vi "output.vi"(8 "error in":errorcluster, 10 "data table in":T1, 11 "JSON_RPC_Interface runtime in":refnum<class "JSON_RPC_Interface runtime.lvclass">) -> (0 "error out":errorcluster, 2 "data table out":T1, 3 "JSON_RPC_Interface runtime out":refnum<class "JSON_RPC_Interface runtime.lvclass">)   [LabVIEW 2017, in "JSON_RPC_Interface runtime.lvclass"]
doc: "Provides an interface for writing data to a module at runtime. While this interface performs no operations, a child should provide an override which may write to any open sessions, references, or interfaces."
uses:
  JSON_RPC_Interface runtime.lvclass
  <vilib>/NI/Tag Bus/table/data table.ctl
  JSON_RPC_Interface runtime.lvclass/JSON_RPC_Interface runtime.ctl
  <vilib>/NI/NI JSONRPC Server Framework/Classes/Request/Request.lvclass/Request.ctl
  <vilib>/NI/Tag Bus/table/data polymorphs/read one/read Double.vi
  <vilib>/NI/Tag Bus/table/data polymorphs/read one/read Single.vi
  <vilib>/NI/Tag Bus/table/data polymorphs/read one/read I64.vi
  <vilib>/NI/Tag Bus/table/data polymorphs/read one/read I32.vi
  <vilib>/NI/Tag Bus/table/data polymorphs/read one/read I16.vi
  <vilib>/NI/Tag Bus/table/data polymorphs/read one/read I8.vi
  <vilib>/NI/Tag Bus/table/data polymorphs/read one/read U64.vi
  <vilib>/NI/Tag Bus/table/data polymorphs/read one/read U32.vi
  <vilib>/NI/Tag Bus/table/data polymorphs/read one/read U16.vi
  <vilib>/NI/Tag Bus/table/data polymorphs/read one/read U8.vi
  <vilib>/NI/Tag Bus/table/data polymorphs/read one/read Boolean.vi
  <vilib>/NI/Tag Bus/table/data polymorphs/read one/read String.vi
  <vilib>/NI/Tag Bus/table/data polymorphs/read one/read Array of Double.vi
  <vilib>/NI/Tag Bus/table/data polymorphs/read one/read Array of Single.vi
  <vilib>/NI/Tag Bus/table/data polymorphs/read one/read Array of I64.vi
  <vilib>/NI/Tag Bus/table/data polymorphs/read one/read Array of I32.vi
  <vilib>/NI/Tag Bus/table/data polymorphs/read one/read Array of I16.vi
  <vilib>/NI/Tag Bus/table/data polymorphs/read one/read Array of I8.vi
  <vilib>/NI/Tag Bus/table/data polymorphs/read one/read Array of U64.vi
  <vilib>/NI/Tag Bus/table/data polymorphs/read one/read Array of U32.vi
  <vilib>/NI/Tag Bus/table/data polymorphs/read one/read Array of U16.vi
  <vilib>/NI/Tag Bus/table/data polymorphs/read one/read Array of U8.vi
  <vilib>/NI/Tag Bus/table/data polymorphs/read one/read Array of Boolean.vi
  <vilib>/NI/Tag Bus/table/data polymorphs/read one/read Array of String.vi
  <vilib>/NI/NI JSONRPC Server Framework/Classes/Request/request.Read params.vi
  <vilib>/NI/NI JSONRPC Server Framework/Classes/params/params.To JSON Tree.vi
  <vilib>/NI/NI JSONRPC Server Framework/Classes/Server/Add Response (Internal Error from Request).vi
  <vilib>/NI/JSON Support for LabVIEW/JSON Value/New JSON Value/New JSON ({String}).vi
  <vilib>/NI/NI JSONRPC Server Framework/Classes/Server/Add Response (Invalid Params from Request).vi
  <vilib>/NI/JSON Support for LabVIEW/JSON Value/Object/Insert Value/Insert Value (Numeric).vi
  <vilib>/NI/JSON Support for LabVIEW/JSON Value/Object/Insert Value/Insert Value (Boolean).vi
  <vilib>/NI/JSON Support for LabVIEW/JSON Value/Object/Insert Value/Insert Value (String).vi
  <vilib>/NI/JSON Support for LabVIEW/JSON Value/Object/Insert Value/Insert Value (Numeric[]).vi
  <vilib>/NI/JSON Support for LabVIEW/JSON Value/Object/Insert Value/Insert Value (Boolean[]).vi
  <vilib>/NI/JSON Support for LabVIEW/JSON Value/Object/Insert Value/Insert Value (String[]).vi
  <vilib>/NI/NI JSONRPC Server Framework/Classes/Server/Add Response (Result from Request).vi
  <vilib>/NI/JSON Support for LabVIEW/JSON Value/JSON Value.lvclass
  <vilib>/NI/Tag Bus/table/data table.lvlib
  <vilib>/NI/NI JSONRPC Server Framework/Classes/Server/JSONRPC Server.lvclass
  <vilib>/NI/NI JSONRPC Server Framework/Classes/Request/Request.lvclass
  <vilib>/NI/JSON Support for LabVIEW/JSON Variant Support/JSON Variant Support.lvclass
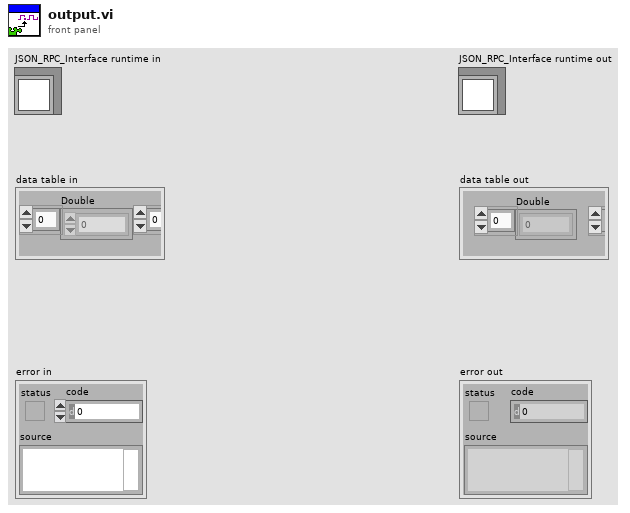
[diagram p1: front panel]
types:
  T1 = typedef "tag bus.lvlib/data table.lvlib/data table.ctl" = cluster{"Double":dbl[], "Single":sgl[], "I64":i64[], "I32":i32[], "I16":i16[], "I8":i8[], "U64":u64[], "U32":u32[], "U16":u16[], "U8":u8[], "Boolean":bool[], "String":string[], "Array of Double":cluster{"DBL Array":dbl[]}[], "Array of Single":cluster{"SGL Array":sgl[]}[], "Array of I64":cluster{"I64 Array":i64[]}[], "Array of I32":cluster{"I32 Array":i32[]}[], "Array of I16":cluster{"I16 Array":i16[]}[], "Array of I8":cluster{"I8 Array":i8[]}[], "Array of U64":cluster{"U64 Array":u64[]}[], "Array of U32":cluster{"U32 Array":u32[]}[], "Array of U16":cluster{"U16 Array":u16[]}[], "Array of U8":cluster{"U8 Array":u8[]}[], "Array of Boolean":cluster{"Boolean Array":bool[]}[], "Array of String":cluster{"String Array":string[]}[]}
  T2 = typedef "tag bus.lvlib/tag descriptor.lvclass/Data Type.ctl" = enum16{"Double", "Single", "I64", "I32", "I16", "I8", "U64", "U32", "U16", "U8", "Boolean", "String", "Array of Double", "Array of Single", "Array of I64", "Array of I32", "Array of I16", "Array of I8", "Array of U64", "Array of U32", "Array of U16", "Array of U8", "Array of Boolean", "Array of String"}
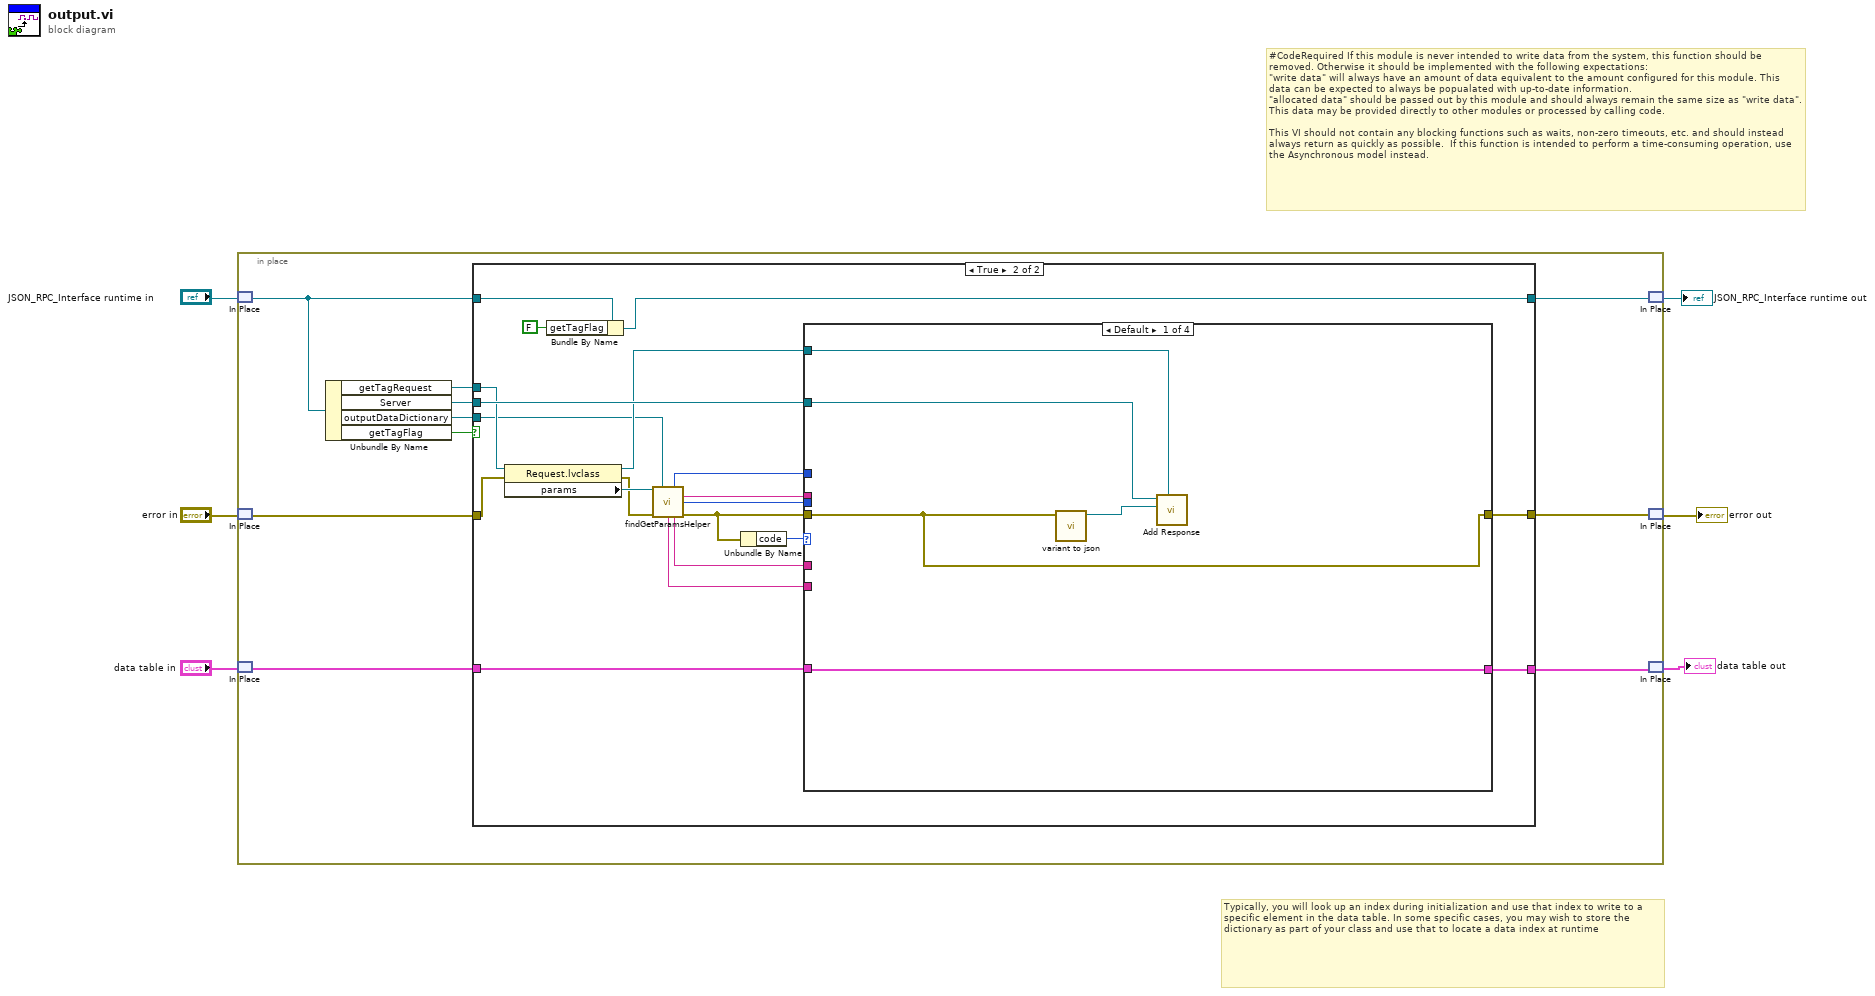
[diagram p0: block diagram]
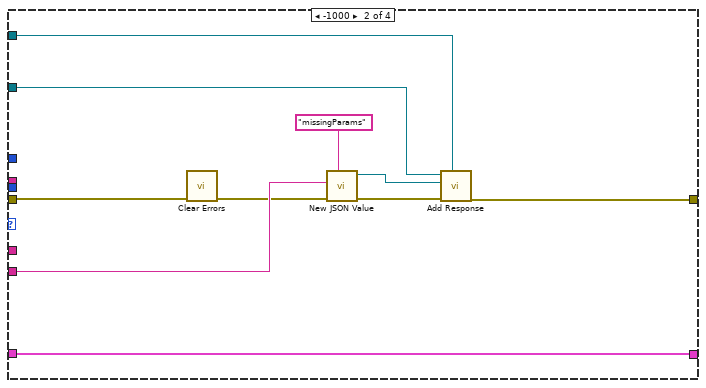
[diagram p3: hidden frame]
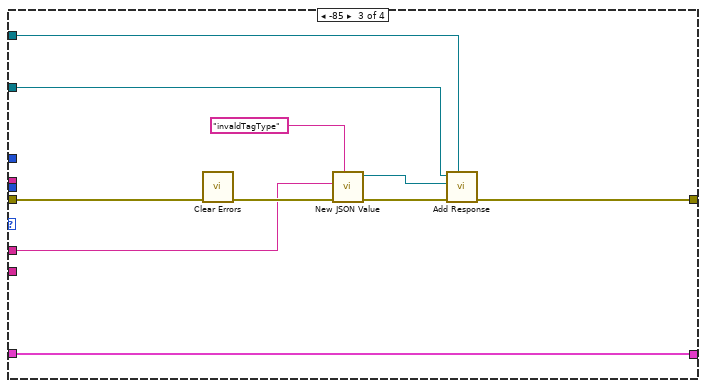
[diagram p4: hidden frame]
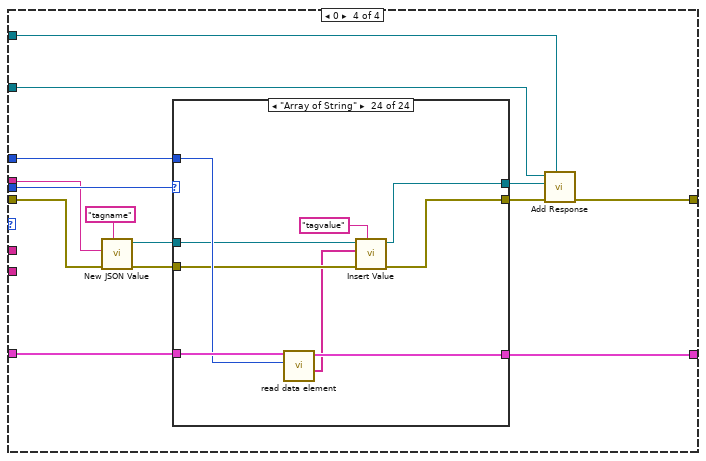
[diagram p5: hidden frame]
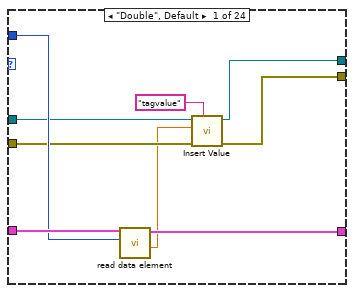
[diagram p6: hidden frame]
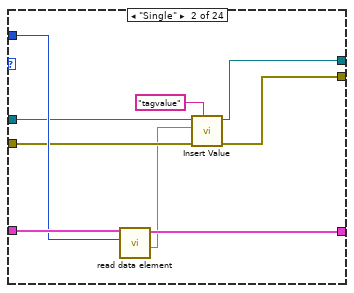
[diagram p7: hidden frame]
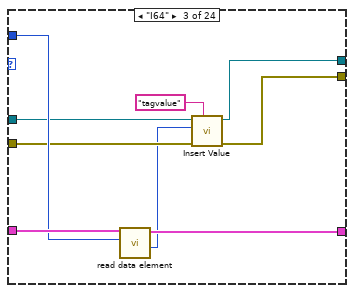
[diagram p8: hidden frame]
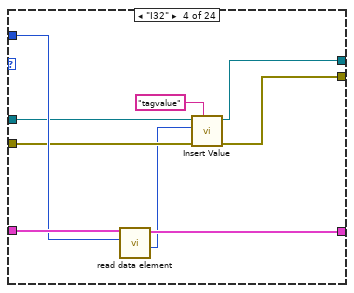
[diagram p9: hidden frame]
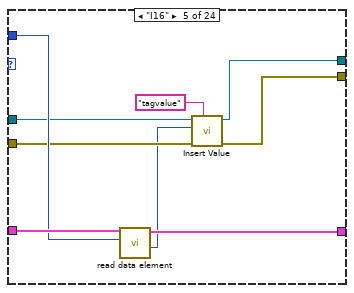
[diagram p10: hidden frame]
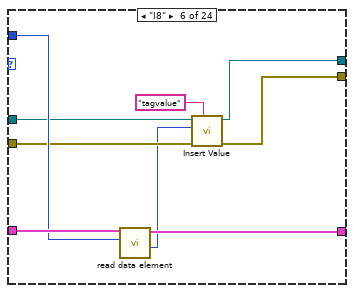
[diagram p11: hidden frame]
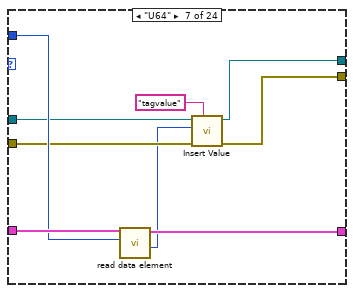
[diagram p12: hidden frame]
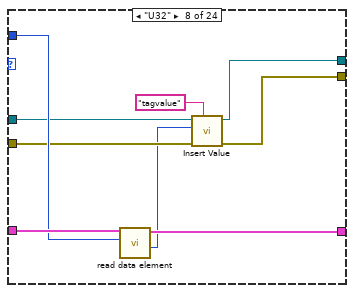
[diagram p13: hidden frame]
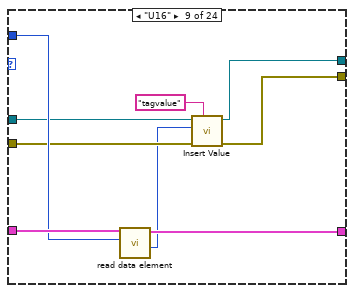
[diagram p14: hidden frame]
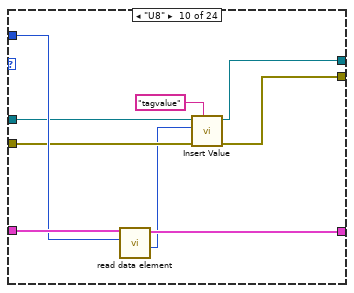
[diagram p15: hidden frame]
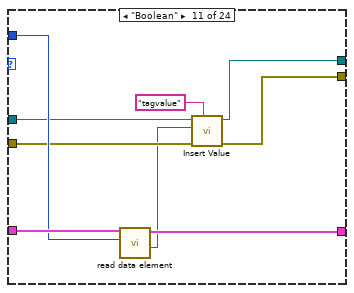
[diagram p16: hidden frame]
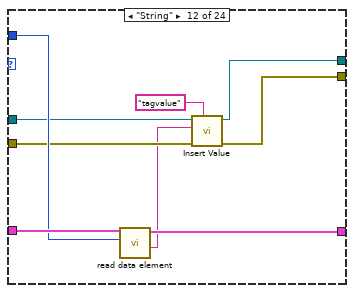
[diagram p17: hidden frame]
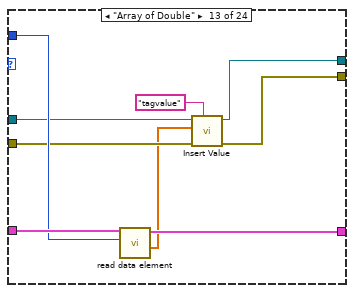
[diagram p18: hidden frame]
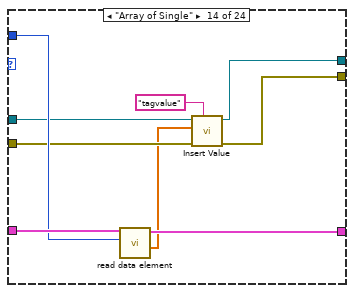
[diagram p19: hidden frame]
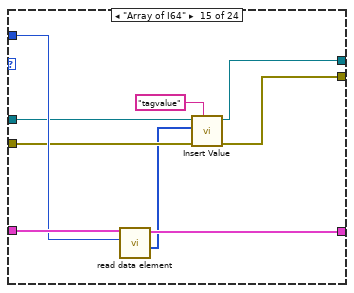
[diagram p20: hidden frame]
diagram:
  # "Typically, you will look up an index during initialization and use that index to write to a specific element in the data table. In some specific cases, you may wish to store the dictionary as part of your class and use that to locate a data index at runtime"
  # "#CodeRequired If this module is never intended to write data from the system, this function should be removed. Otherwise it should be implemented with the following expectations:\n\"write data\" will always have an amount of data equivalent to the amount configured for this module. This data can be expected to always be popualated with up-to-date information.\n\"allocated data\" should be passed out by this module and should always remain the same size as \"write data\". This data may be provided directly to other modules or processed by calling code.\n\nThis VI should not contain any blocking functions such as waits, non-zero timeouts, etc. and should instead always return as quickly as possible.  If this function is intended to perform a time-consuming operation, use the Asynchronous model instead."
  n1 = in-place {
    n2 = in-place-match #1("JSON_RPC_Interface runtime in") -> (w8:refnum<class "JSON_RPC_Interface runtime.lvclass">)
    n3 = in-place-match #2("error in") -> (w11:errorcluster)
    n4 = in-place-match #3("data table in") -> (w16:T1)
    n5 = Unbundle By Name(w8) -> ("getTagRequest"=w12:refnum<class "Request.lvclass">, "Server"=w13:refnum<class "JSONRPC Server.lvclass">, "outputDataDictionary"=w10:refnum<class "data dictionary.lvclass">, "getTagFlag"=w9:bool)
    n6 = case shown="True" w9 {
      tunnel: w16 -> [w19 w38]
      tunnel: [w19 w37] -> w15
      tunnel: [w18 w36] -> w14
      tunnel: w13 -> [_ w35]
      tunnel: w12 -> [_ w34]
      tunnel: w11 -> [w18 w32]
      tunnel: w10 -> [_ w30]
      tunnel: w8 -> [w17 w22]
      tunnel: [w17 w20] -> w7
      frame False {
      }
      frame True {
        n7 = property class="Request.lvclass"(reference=w34, error in=w32) -> (reference out=w33:refnum<class "Request.lvclass">, error out=w29:errorcluster, "params"=w31:refnum<class "JSON Value.lvclass">)
        n8 = Bundle By Name(cluster=w22, "getTagFlag"=FALSE) -> (w20:refnum<class "JSON_RPC_Interface runtime.lvclass">)
        n9 = call "findGetParamsHelper.vi"("params in"=w31, "outputDataDictionary"=w30, "error in"=w29) -> ("tagindex"=w23:i32, "tagname"=w25:string, "tagtype"=w24:T2, "missingParam"=w26:string, "invalidTagType"=w27:string, "error out"=w28:errorcluster)  [unwired: 6 in, 1 out]
        n10 = Unbundle By Name(w28) -> ("code"=w39:i32)
        n11 = case shown="Default" w39 {
          tunnel: w38 -> [w44 w54 w64 w78]
          tunnel: [w44 w54 w64 w77] -> w37
          tunnel: [w41 w50 w58 w65] -> w36
          tunnel: w35 -> [w42 w49 w56 w66]
          tunnel: w33 -> [w43 w48 w57 w74]
          tunnel: w28 -> [w41 w45 w59 w73]
          tunnel: w27 -> [_ _ w55 _]
          tunnel: w26 -> [_ w47 _ _]
          tunnel: w25 -> [_ _ _ w70]
          tunnel: w24 -> [_ _ _ w76]
          tunnel: w23 -> [_ _ _ w75]
          frame Default {
            n12 = call <vilib>:"variant to json.vi"("Variant"=w41) -> ("JSON Value"=w40:refnum<class "JSON Value.lvclass">)  [unwired: 9 in, 1 out]
            n13 = call-poly <vilib>:"Add Response.vi"("Request"=w43, "data"=w40, "Server in"=w42) -> ()  [unwired: 6 in, 3 out]
          }
          frame -1000 {
            n14 = call <vilib>:"Clear Errors.vi"("error in (no error)"=w45) -> ("error out"=w46:errorcluster)  [unwired: 5 in, 1 out]
            n15 = call-poly <vilib>:"New JSON Value.vi"("key"="missingParams", "error in (no error)"=w46, "value"=w47) -> ("error out"=w52:errorcluster, "JSON Value out"=w51:refnum<class "JSON Value.lvclass">)  [unwired: 7 in]
            n16 = call-poly <vilib>:"Add Response.vi"("Request"=w48, "error in (no error)"=w52, "data"=w51, "Server in"=w49) -> ("error out"=w50:errorcluster)  [unwired: 5 in, 2 out]
          }
          frame -85 {
            n17 = call <vilib>:"Clear Errors.vi"("error in (no error)"=w59) -> ("error out"=w61:errorcluster)  [unwired: 5 in, 1 out]
            n18 = call-poly <vilib>:"New JSON Value.vi"("key"="invaldTagType", "error in (no error)"=w61, "value"=w55) -> ("error out"=w63:errorcluster, "JSON Value out"=w62:refnum<class "JSON Value.lvclass">)  [unwired: 7 in]
            n19 = call-poly <vilib>:"Add Response.vi"("Request"=w57, "error in (no error)"=w63, "data"=w62, "Server in"=w56) -> ("error out"=w58:errorcluster)  [unwired: 5 in, 2 out]
          }
          frame 0 {
            n20 = call-poly <vilib>:"New JSON Value.vi"("key"="tagname", "error in (no error)"=w73, "value"=w70) -> ("error out"=w71:errorcluster, "JSON Value out"=w69:refnum<class "JSON Value.lvclass">)  [unwired: 7 in]
            n21 = case shown="\"Array of String\"" w76 {
              tunnel: w78 -> [w87 w96 w105 w114 w123 w132 w141 w150 w159 w168 w177 w186 w195 w204 w213 w222 w231 w240 w249 w258 w267 w276 w285 w294]
              tunnel: [w86 w95 w104 w113 w122 w131 w140 w149 w158 w167 w176 w185 w194 w203 w212 w221 w230 w239 w248 w257 w266 w275 w284 w293] -> w77
              tunnel: w71 -> [w82 w91 w100 w109 w118 w127 w136 w145 w154 w163 w172 w181 w190 w199 w208 w217 w226 w235 w244 w253 w262 w271 w280 w289]
              tunnel: w75 -> [w85 w94 w103 w112 w121 w130 w139 w148 w157 w166 w175 w184 w193 w202 w211 w220 w229 w238 w247 w256 w265 w274 w283 w292]
              tunnel: w69 -> [w84 w93 w102 w111 w120 w129 w138 w147 w156 w165 w174 w183 w192 w201 w210 w219 w228 w237 w246 w255 w264 w273 w282 w291]
              tunnel: [w80 w89 w98 w107 w116 w125 w134 w143 w152 w161 w170 w179 w188 w197 w206 w215 w224 w233 w242 w251 w260 w269 w278 w287] -> w68
              tunnel: [w79 w88 w97 w106 w115 w124 w133 w142 w151 w160 w169 w178 w187 w196 w205 w214 w223 w232 w241 w250 w259 w268 w277 w286] -> w67
              frame "Double", Default {
                n22 = call-poly <vilib>:"read data element.vi"("index"=w85, "data table in"=w87) -> ("value"=w81:dbl, "data table out"=w86:T1)  [unwired: 8 in]
                n23 = call-poly <vilib>:"Insert Value.vi"("key"="tagvalue", "error in (no error)"=w82, "value"=w81, "JSON Value in"=w84) -> ("error out"=w80:errorcluster, "JSON Value out"=w79:refnum<class "JSON Value.lvclass">)  [unwired: 5 in, 1 out]
              }
              frame "Single" {
                n24 = call-poly <vilib>:"read data element.vi"("index"=w94, "data table in"=w96) -> ("value"=w90:sgl, "data table out"=w95:T1)  [unwired: 8 in]
                n25 = call-poly <vilib>:"Insert Value.vi"("key"="tagvalue", "error in (no error)"=w91, "value"=w90, "JSON Value in"=w93) -> ("error out"=w89:errorcluster, "JSON Value out"=w88:refnum<class "JSON Value.lvclass">)  [unwired: 5 in, 1 out]
              }
              frame "I64" {
                n26 = call-poly <vilib>:"read data element.vi"("index"=w103, "data table in"=w105) -> ("value"=w99:i64, "data table out"=w104:T1)  [unwired: 8 in]
                n27 = call-poly <vilib>:"Insert Value.vi"("key"="tagvalue", "error in (no error)"=w100, "value"=w99, "JSON Value in"=w102) -> ("error out"=w98:errorcluster, "JSON Value out"=w97:refnum<class "JSON Value.lvclass">)  [unwired: 5 in, 1 out]
              }
              frame "I32" {
                n28 = call-poly <vilib>:"read data element.vi"("index"=w112, "data table in"=w114) -> ("value"=w108:i32, "data table out"=w113:T1)  [unwired: 8 in]
                n29 = call-poly <vilib>:"Insert Value.vi"("key"="tagvalue", "error in (no error)"=w109, "value"=w108, "JSON Value in"=w111) -> ("error out"=w107:errorcluster, "JSON Value out"=w106:refnum<class "JSON Value.lvclass">)  [unwired: 5 in, 1 out]
              }
              frame "I16" {
                n30 = call-poly <vilib>:"read data element.vi"("index"=w121, "data table in"=w123) -> ("value"=w117:i16, "data table out"=w122:T1)  [unwired: 8 in]
                n31 = call-poly <vilib>:"Insert Value.vi"("key"="tagvalue", "error in (no error)"=w118, "value"=w117, "JSON Value in"=w120) -> ("error out"=w116:errorcluster, "JSON Value out"=w115:refnum<class "JSON Value.lvclass">)  [unwired: 5 in, 1 out]
              }
              frame "I8" {
                n32 = call-poly <vilib>:"read data element.vi"("index"=w130, "data table in"=w132) -> ("value"=w126:i8, "data table out"=w131:T1)  [unwired: 8 in]
                n33 = call-poly <vilib>:"Insert Value.vi"("key"="tagvalue", "error in (no error)"=w127, "value"=w126, "JSON Value in"=w129) -> ("error out"=w125:errorcluster, "JSON Value out"=w124:refnum<class "JSON Value.lvclass">)  [unwired: 5 in, 1 out]
              }
              frame "U64" {
                n34 = call-poly <vilib>:"read data element.vi"("index"=w139, "data table in"=w141) -> ("value"=w135:u64, "data table out"=w140:T1)  [unwired: 8 in]
                n35 = call-poly <vilib>:"Insert Value.vi"("key"="tagvalue", "error in (no error)"=w136, "value"=w135, "JSON Value in"=w138) -> ("error out"=w134:errorcluster, "JSON Value out"=w133:refnum<class "JSON Value.lvclass">)  [unwired: 5 in, 1 out]
              }
              frame "U32" {
                n36 = call-poly <vilib>:"read data element.vi"("index"=w148, "data table in"=w150) -> ("value"=w144:u32, "data table out"=w149:T1)  [unwired: 8 in]
                n37 = call-poly <vilib>:"Insert Value.vi"("key"="tagvalue", "error in (no error)"=w145, "value"=w144, "JSON Value in"=w147) -> ("error out"=w143:errorcluster, "JSON Value out"=w142:refnum<class "JSON Value.lvclass">)  [unwired: 5 in, 1 out]
              }
              frame "U16" {
                n38 = call-poly <vilib>:"read data element.vi"("index"=w157, "data table in"=w159) -> ("value"=w153:u16, "data table out"=w158:T1)  [unwired: 8 in]
                n39 = call-poly <vilib>:"Insert Value.vi"("key"="tagvalue", "error in (no error)"=w154, "value"=w153, "JSON Value in"=w156) -> ("error out"=w152:errorcluster, "JSON Value out"=w151:refnum<class "JSON Value.lvclass">)  [unwired: 5 in, 1 out]
              }
              frame "U8" {
                n40 = call-poly <vilib>:"read data element.vi"("index"=w166, "data table in"=w168) -> ("value"=w162:u8, "data table out"=w167:T1)  [unwired: 8 in]
                n41 = call-poly <vilib>:"Insert Value.vi"("key"="tagvalue", "error in (no error)"=w163, "value"=w162, "JSON Value in"=w165) -> ("error out"=w161:errorcluster, "JSON Value out"=w160:refnum<class "JSON Value.lvclass">)  [unwired: 5 in, 1 out]
              }
              frame "Boolean" {
                n42 = call-poly <vilib>:"read data element.vi"("index"=w175, "data table in"=w177) -> ("value"=w171:bool, "data table out"=w176:T1)  [unwired: 8 in]
                n43 = call-poly <vilib>:"Insert Value.vi"("key"="tagvalue", "error in (no error)"=w172, "value"=w171, "JSON Value in"=w174) -> ("error out"=w170:errorcluster, "JSON Value out"=w169:refnum<class "JSON Value.lvclass">)  [unwired: 5 in, 1 out]
              }
              frame "String" {
                n44 = call-poly <vilib>:"read data element.vi"("index"=w184, "data table in"=w186) -> ("value"=w180:string, "data table out"=w185:T1)  [unwired: 8 in]
                n45 = call-poly <vilib>:"Insert Value.vi"("key"="tagvalue", "error in (no error)"=w181, "value"=w180, "JSON Value in"=w183) -> ("error out"=w179:errorcluster, "JSON Value out"=w178:refnum<class "JSON Value.lvclass">)  [unwired: 5 in, 1 out]
              }
              frame "Array of Double" {
                n46 = call-poly <vilib>:"read data element.vi"("index"=w193, "data table in"=w195) -> ("value"=w189:dbl[], "data table out"=w194:T1)  [unwired: 8 in]
                n47 = call-poly <vilib>:"Insert Value.vi"("key"="tagvalue", "error in (no error)"=w190, "JSON Data in"=w189, "JSON Value in"=w192) -> ("error out"=w188:errorcluster, "JSON Value out"=w187:refnum<class "JSON Value.lvclass">)  [unwired: 5 in, 1 out]
              }
              frame "Array of Single" {
                n48 = call-poly <vilib>:"read data element.vi"("index"=w202, "data table in"=w204) -> ("value"=w198:sgl[], "data table out"=w203:T1)  [unwired: 8 in]
                n49 = call-poly <vilib>:"Insert Value.vi"("key"="tagvalue", "error in (no error)"=w199, "JSON Data in"=w198, "JSON Value in"=w201) -> ("error out"=w197:errorcluster, "JSON Value out"=w196:refnum<class "JSON Value.lvclass">)  [unwired: 5 in, 1 out]
              }
              frame "Array of I64" {
                n50 = call-poly <vilib>:"read data element.vi"("index"=w211, "data table in"=w213) -> ("value"=w207:i64[], "data table out"=w212:T1)  [unwired: 8 in]
                n51 = call-poly <vilib>:"Insert Value.vi"("key"="tagvalue", "error in (no error)"=w208, "JSON Data in"=w207, "JSON Value in"=w210) -> ("error out"=w206:errorcluster, "JSON Value out"=w205:refnum<class "JSON Value.lvclass">)  [unwired: 5 in, 1 out]
              }
              frame "Array of I32" {
                n52 = call-poly <vilib>:"read data element.vi"("index"=w220, "data table in"=w222) -> ("value"=w216:i32[], "data table out"=w221:T1)  [unwired: 8 in]
                n53 = call-poly <vilib>:"Insert Value.vi"("key"="tagvalue", "error in (no error)"=w217, "JSON Data in"=w216, "JSON Value in"=w219) -> ("error out"=w215:errorcluster, "JSON Value out"=w214:refnum<class "JSON Value.lvclass">)  [unwired: 5 in, 1 out]
              }
              frame "Array of I16" {
                n54 = call-poly <vilib>:"read data element.vi"("index"=w229, "data table in"=w231) -> ("value"=w225:i16[], "data table out"=w230:T1)  [unwired: 8 in]
                n55 = call-poly <vilib>:"Insert Value.vi"("key"="tagvalue", "error in (no error)"=w226, "JSON Data in"=w225, "JSON Value in"=w228) -> ("error out"=w224:errorcluster, "JSON Value out"=w223:refnum<class "JSON Value.lvclass">)  [unwired: 5 in, 1 out]
              }
              frame "Array of I8" {
                n56 = call-poly <vilib>:"read data element.vi"("index"=w238, "data table in"=w240) -> ("value"=w234:i8[], "data table out"=w239:T1)  [unwired: 8 in]
                n57 = call-poly <vilib>:"Insert Value.vi"("key"="tagvalue", "error in (no error)"=w235, "JSON Data in"=w234, "JSON Value in"=w237) -> ("error out"=w233:errorcluster, "JSON Value out"=w232:refnum<class "JSON Value.lvclass">)  [unwired: 5 in, 1 out]
              }
              frame "Array of U64" {
                n58 = call-poly <vilib>:"read data element.vi"("index"=w247, "data table in"=w249) -> ("value"=w243:u64[], "data table out"=w248:T1)  [unwired: 8 in]
                n59 = call-poly <vilib>:"Insert Value.vi"("key"="tagvalue", "error in (no error)"=w244, "JSON Data in"=w243, "JSON Value in"=w246) -> ("error out"=w242:errorcluster, "JSON Value out"=w241:refnum<class "JSON Value.lvclass">)  [unwired: 5 in, 1 out]
              }
              frame "Array of U32" {
                n60 = call-poly <vilib>:"read data element.vi"("index"=w256, "data table in"=w258) -> ("value"=w252:u32[], "data table out"=w257:T1)  [unwired: 8 in]
                n61 = call-poly <vilib>:"Insert Value.vi"("key"="tagvalue", "error in (no error)"=w253, "JSON Data in"=w252, "JSON Value in"=w255) -> ("error out"=w251:errorcluster, "JSON Value out"=w250:refnum<class "JSON Value.lvclass">)  [unwired: 5 in, 1 out]
              }
              frame "Array of U16" {
                n62 = call-poly <vilib>:"read data element.vi"("index"=w265, "data table in"=w267) -> ("value"=w261:u16[], "data table out"=w266:T1)  [unwired: 8 in]
                n63 = call-poly <vilib>:"Insert Value.vi"("key"="tagvalue", "error in (no error)"=w262, "JSON Data in"=w261, "JSON Value in"=w264) -> ("error out"=w260:errorcluster, "JSON Value out"=w259:refnum<class "JSON Value.lvclass">)  [unwired: 5 in, 1 out]
              }
              frame "Array of U8" {
                n64 = call-poly <vilib>:"read data element.vi"("index"=w274, "data table in"=w276) -> ("value"=w270:u8[], "data table out"=w275:T1)  [unwired: 8 in]
                n65 = call-poly <vilib>:"Insert Value.vi"("key"="tagvalue", "error in (no error)"=w271, "JSON Data in"=w270, "JSON Value in"=w273) -> ("error out"=w269:errorcluster, "JSON Value out"=w268:refnum<class "JSON Value.lvclass">)  [unwired: 5 in, 1 out]
              }
              frame "Array of Boolean" {
                n66 = call-poly <vilib>:"read data element.vi"("index"=w283, "data table in"=w285) -> ("value"=w279:bool[], "data table out"=w284:T1)  [unwired: 8 in]
                n67 = call-poly <vilib>:"Insert Value.vi"("key"="tagvalue", "error in (no error)"=w280, "JSON Data in"=w279, "JSON Value in"=w282) -> ("error out"=w278:errorcluster, "JSON Value out"=w277:refnum<class "JSON Value.lvclass">)  [unwired: 5 in, 1 out]
              }
              frame "Array of String" {
                n68 = call-poly <vilib>:"read data element.vi"("index"=w292, "data table in"=w294) -> ("value"=w288:string[], "data table out"=w293:T1)  [unwired: 8 in]
                n69 = call-poly <vilib>:"Insert Value.vi"("key"="tagvalue", "error in (no error)"=w289, "JSON Data in"=w288, "JSON Value in"=w291) -> ("error out"=w287:errorcluster, "JSON Value out"=w286:refnum<class "JSON Value.lvclass">)  [unwired: 5 in, 1 out]
              }
            }
            n70 = call-poly <vilib>:"Add Response.vi"("Request"=w74, "error in (no error)"=w68, "JSON Value in"=w67, "Server in"=w66) -> ("error out"=w65:errorcluster)  [unwired: 5 in, 2 out]
          }
        }
      }
    }
    n71 = in-place-match #1(w7) -> (→"JSON_RPC_Interface runtime out":refnum<class "JSON_RPC_Interface runtime.lvclass">)
    n72 = in-place-match #2(w14) -> (→"error out":errorcluster)
    n73 = in-place-match #3(w15) -> (→"data table out":T1)
  }
